vi "Vision Processing.vi"(4 "error in (no error)":errorcluster, 7 "Image Size":T9=enum."320x240") -> ()   [LabVIEW 2015]
doc: "This VI runs in parallel to other tasks. It gets images from the camera, processes them for color or shape and use that information to affect robot behavior."
uses:
  <vilib>/Rock Robotics/WPI/Camera/WPI_CameraImageSize.ctl
  <vilib>/vision/Measure.llb/Straight Edge Options.ctl
  <vilib>/vision/Measure.llb/Straight Edge Process.ctl
  <vilib>/vision/Measure.llb/Edge Options.ctl
  <vilib>/vision/Measure.llb/Edge Polarity.ctl
  <vilib>/Rock Robotics/WPI/Camera/WPI_CameraWhite Balance Values.ctl
  <vilib>/Rock Robotics/WPI/Camera/WPI_CameraExposure Values.ctl
  <vilib>/Rock Robotics/WPI/Camera/WPI_CameraFrameRate.ctl
  Robot Global Data.vi
  <vilib>/vision/NI_Vision_Development_Module.lvlib
panel:
  in  "Options":T3={"Search Direction"=0, "Edge Options"={"Edge Polarity"=0, "Kernel Size"=3, "Width"=3, "Minimum Edge Strength"=10.0, "Interpolation Type"=enum."Bilinear Fixed", "Data Processing Method"=enum."Average"}, "Show Search Area"=FALSE, "Show Search Lines"=FALSE, "Show Edges Found"=FALSE, "Show Result"=TRUE, "Search Area Color"=65280, "Search Lines Color"=255, "Edge Locations Color"=16776960, "Result Color"=16711680, "Overlay Group Name"=""} {"Edge Options"."Edge Polarity" items=["All Edges", "Rising Edges", "Falling Edges"]; "Edge Options"."Minimum Edge Strength" format="%.2f"; "Edge Options"."Width" step=2; "Edge Options"."Kernel Size" step=2; "Search Direction" items=["Left to Right", "Right to Left", "Top to Bottom", "Bottom to Top"]}
  out "Image Dst Out":T4(plugin-control)
  out "Corner Point Coordinates[0]":cluster{"X":sgl, "Y":sgl}
  out "Point2 (Pixels)":cluster{"X":sgl, "Y":sgl}
  out "Point1 (Pixels)":cluster{"X":sgl, "Y":sgl}
  in  "Line Fit Options":T5={"Number of Lines"=1, "Type"=enum."First Edge Rake", "Min. Score"=10.0, "Max. Score"=1000.0, "Orientation"=0.0, "Angle Range"=45.0, "Angle Tolerance"=1.0, "Step Size"=7, "Min. SNR (db)"=0.0, "Min. Points (%)"=25.0, "Hough Iterations"=5} {"Min. Points (%)" min=0.0 max=100.0; "Min. SNR (db)" min=0.0; "Max. Score" min=0.0 max=1024.0; "Min. Score" min=0.0 max=1024.0 step=1.0}
  in  "Coordinate System":T7 {"Measurement System"."Axis Reference" items=["Direct", "Indirect"]; "Measurement System"."Angle (deg)" format="%.2f"; "Measurement System"."Origin"."Y" format="%.2f"; "Measurement System"."Origin"."X" format="%.2f"; "Reference System"."Axis Reference" items=["Direct", "Indirect"]; "Reference System"."Angle (deg)" format="%.2f"; "Reference System"."Origin"."Y" format="%.2f"; "Reference System"."Origin"."X" format="%.2f"}
  in  "ROI Descriptor":T8 {"Contours"."Type" items=["No Selection", "Point", "Line", "Rectangle", "Oval", "Polygon", "Free", "Annulus", "Unused2", "Unused3", "Broken Line", "Free Hand Line", "Rotated Rectangle"]}
  out "Center of Mass":cluster{"X":dbl, "Y":dbl}
  out "Calibration Valid":bool[](array[boolean])
  out "max index(es)":i32[](array[numeric])
  out "max value":u8
  in  "Range":cluster{"Lower value":i32, "Upper value":i32}={"Lower value"=240, "Upper value"=255}
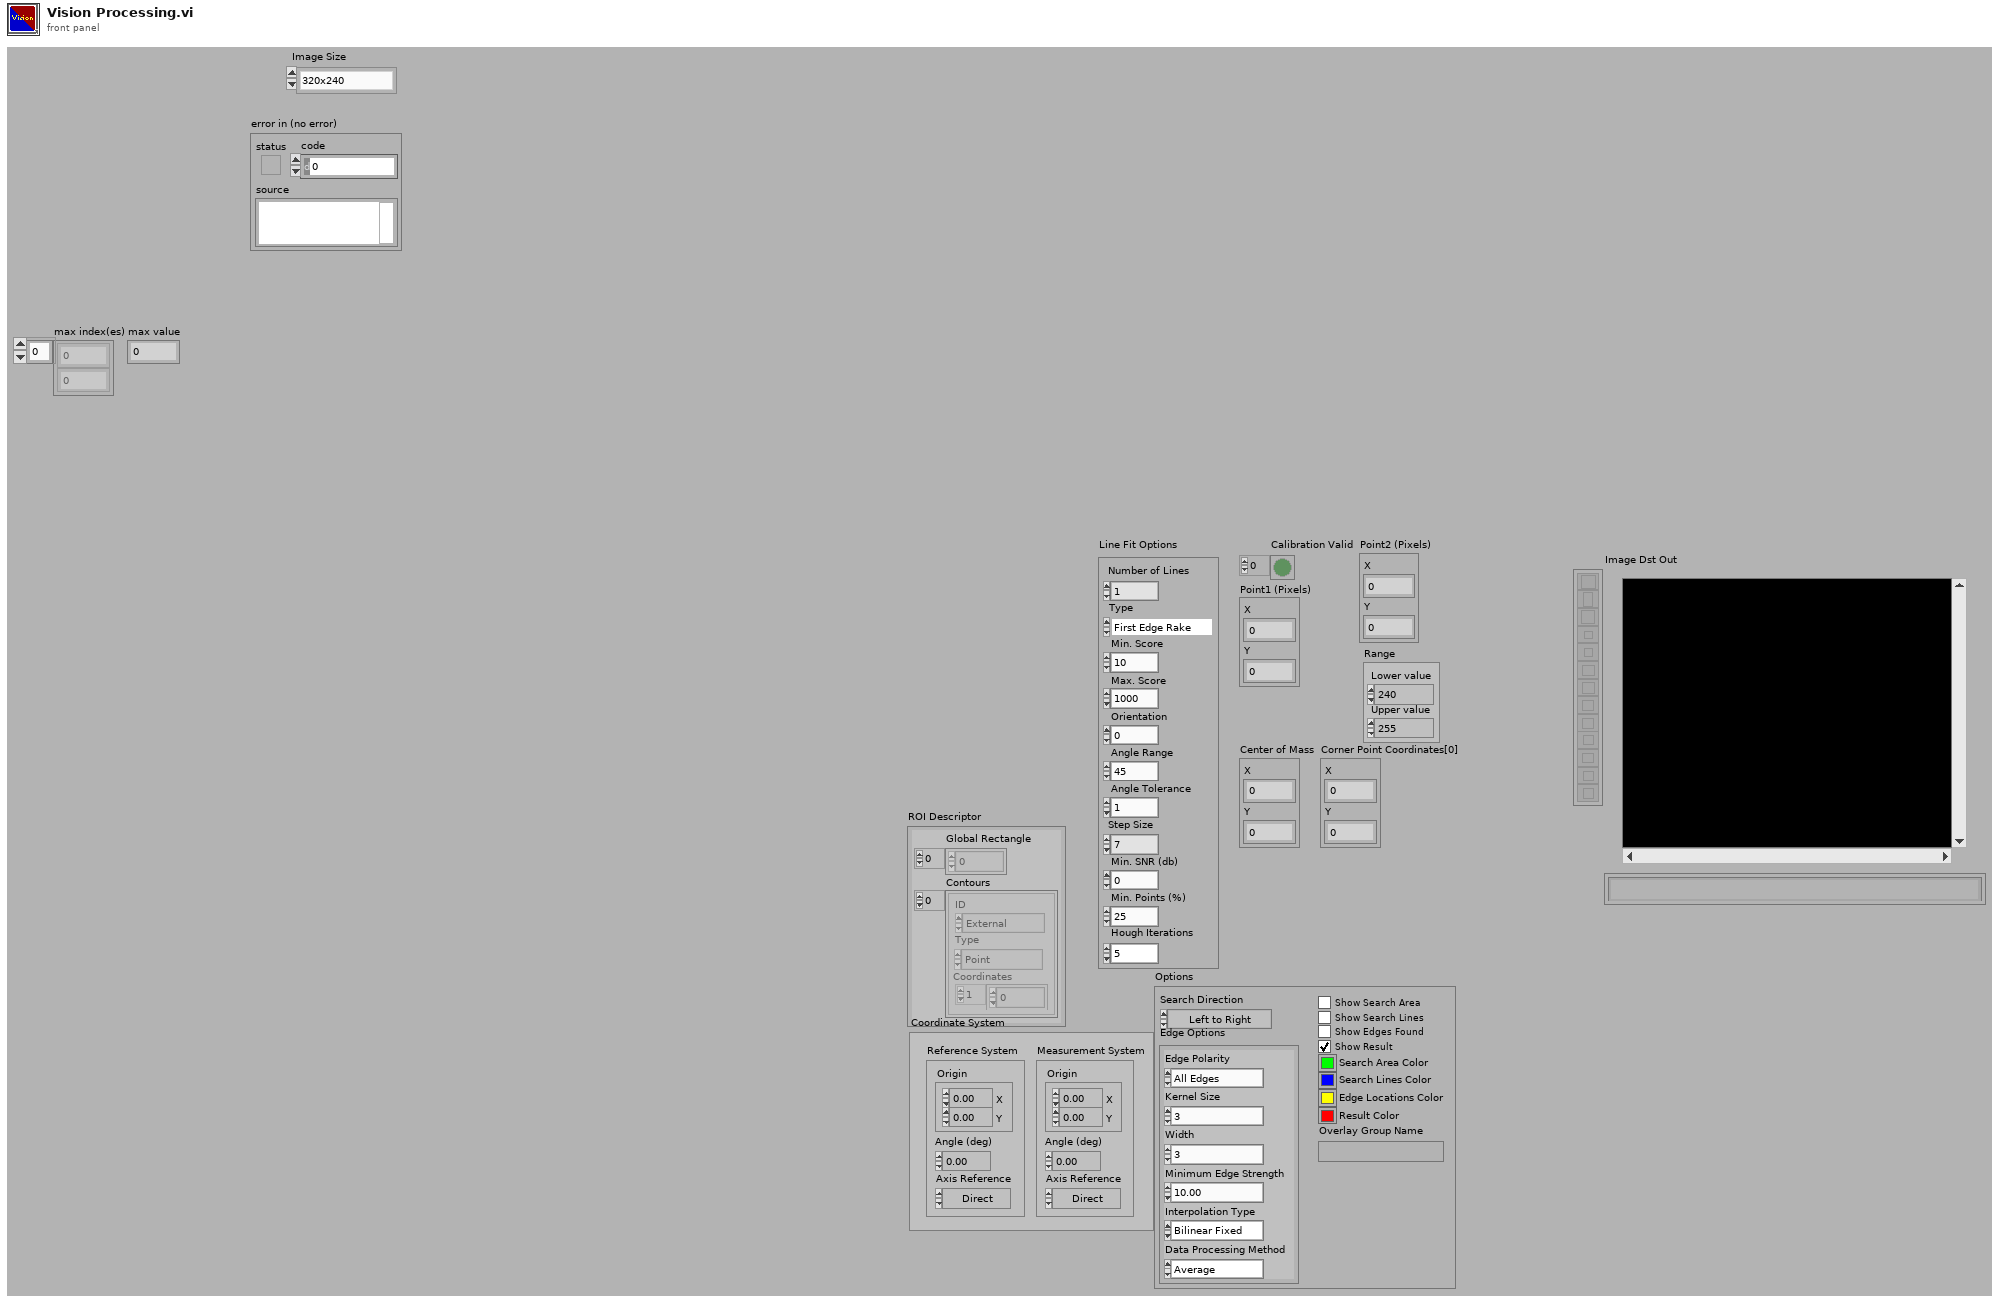
[diagram p1: front panel]
types:
  T1 = typedef "Edge Options.ctl" = cluster{"Edge Polarity":T2, "Kernel Size":u32, "Width":u32, "Minimum Edge Strength":sgl, "Interpolation Type":enum32{"Zero Order", "Bilinear", "Quadratic", "Cubic", "Bilinear Fixed"}, "Data Processing Method":enum32{"Average", "Median"}}
  T2 = typedef "Edge Polarity.ctl" = u32
  T3 = cluster{"Search Direction":u32, "Edge Options":T1, "Show Search Area":bool, "Show Search Lines":bool, "Show Edges Found":bool, "Show Result":bool, "Search Area Color":u32, "Search Lines Color":u32, "Edge Locations Color":u32, "Result Color":u32, "Overlay Group Name":string}
  T4 = typedef "IMAQ Image.ctl" = refnum<image>
  T5 = typedef "Straight Edge Options.ctl" = cluster{"Number of Lines":i32, "Type":T6, "Min. Score":dbl, "Max. Score":dbl, "Orientation":dbl, "Angle Range":dbl, "Angle Tolerance":dbl, "Step Size":u32, "Min. SNR (db)":dbl, "Min. Points (%)":dbl, "Hough Iterations":i32}
  T6 = typedef "Straight Edge Process.ctl" = enum32{"First Edge Rake", "Best Edge Rake", "Hough Edge Rake", "First Edge Projection", "Best Edge Projection"}
  T7 = typedef "IMAQ Coordinate System" = cluster{"Reference System":cluster{"Origin":cluster{"X":sgl, "Y":sgl}, "Angle (deg)":sgl, "Axis Reference":u32}, "Measurement System":cluster{"Origin":cluster{"X":sgl, "Y":sgl}, "Angle (deg)":sgl, "Axis Reference":u32}}
  T8 = cluster{"Global Rectangle":i32[], "Contours":cluster{"ID":enum32{"External", "Internal"}, "Type":u32, "Coordinates":i32[]}[]}
  T9 = typedef "WPI_CameraImageSize.ctl" = enum16{"640x480", "320x240", "160x120", "Custom"}
  T10 = typedef "Image Type" = u32
  T11 = typedef "WPI_CameraFrameRate.ctl" = u32
  T12 = typedef "WPI_CameraExposure Values.ctl" = enum16{"Auto", "Flicker-free 50 Hz", "Flicker-free 60 Hz", "Hold current", "Custom"}
  T13 = typedef "WPI_CameraWhite Balance Values.ctl" = enum16{"Auto", "Fixed indoor", "Fixed outdoor 1", "Fixed outdoor 2", "Fixed fluorescent 1", "Fixed fluorescent 2", "Hold current", "Custom"}
  T14 = typedef "WPI_CameraDevRef.ctl" = cluster{"Camera Address":string, "CameraStatus":errorcluster}
  T15 = enum32{"AutoM", "Close", "Dilate", "Erode", "Gradient", "Gradient out", "Gradient in", "Hit miss", "Open", "PClose", "POpen", "Thick", "Thin"}
  T16 = cluster{"Area":dbl, "Number of Holes":dbl, "Bounding Rect":cluster{"Left":dbl, "Top":dbl, "Right":dbl, "Bottom":dbl}, "Center of Mass":cluster{"X":dbl, "Y":dbl}, "Orientation":dbl, "Dimensions":cluster{"Width":dbl, "Height":dbl}}[]
  T17 = cluster{"Point1 (Pixels)":cluster{"X":sgl, "Y":sgl}, "Point2 (Pixels)":cluster{"X":sgl, "Y":sgl}, "Point1 (Real-World)":cluster{"X":sgl, "Y":sgl}, "Point2 (Real-World)":cluster{"X":sgl, "Y":sgl}, "Angle (Pixel)":dbl, "Angle (Real-World)":dbl, "Score":dbl, "Straightness":dbl, "Average SNR (db)":dbl, "Calibration Valid":bool}[]
  T18 = cluster{"Particle Reports (Pixels)[0]":cluster{"Area":dbl, "Number of Holes":dbl, "Bounding Rect":cluster{"Left":dbl, "Top":dbl, "Right":dbl, "Bottom":dbl}, "Center of Mass":cluster{"X":dbl, "Y":dbl}, "Orientation":dbl, "Dimensions":cluster{"Width":dbl, "Height":dbl}}, "Particle Reports (Pixels)[1]":cluster{"Area":dbl, "Number of Holes":dbl, "Bounding Rect":cluster{"Left":dbl, "Top":dbl, "Right":dbl, "Bottom":dbl}, "Center of Mass":cluster{"X":dbl, "Y":dbl}, "Orientation":dbl, "Dimensions":cluster{"Width":dbl, "Height":dbl}}, "Particle Reports (Pixels)[2]":cluster{"Area":dbl, "Number of Holes":dbl, "Bounding Rect":cluster{"Left":dbl, "Top":dbl, "Right":dbl, "Bottom":dbl}, "Center of Mass":cluster{"X":dbl, "Y":dbl}, "Orientation":dbl, "Dimensions":cluster{"Width":dbl, "Height":dbl}}, "Particle Reports (Pixels)[3]":cluster{"Area":dbl, "Number of Holes":dbl, "Bounding Rect":cluster{"Left":dbl, "Top":dbl, "Right":dbl, "Bottom":dbl}, "Center of Mass":cluster{"X":dbl, "Y":dbl}, "Orientation":dbl, "Dimensions":cluster{"Width":dbl, "Height":dbl}}, "Particle Reports (Pixels)[4]":cluster{"Area":dbl, "Number of Holes":dbl, "Bounding Rect":cluster{"Left":dbl, "Top":dbl, "Right":dbl, "Bottom":dbl}, "Center of Mass":cluster{"X":dbl, "Y":dbl}, "Orientation":dbl, "Dimensions":cluster{"Width":dbl, "Height":dbl}}, "Particle Reports (Pixels)[5]":cluster{"Area":dbl, "Number of Holes":dbl, "Bounding Rect":cluster{"Left":dbl, "Top":dbl, "Right":dbl, "Bottom":dbl}, "Center of Mass":cluster{"X":dbl, "Y":dbl}, "Orientation":dbl, "Dimensions":cluster{"Width":dbl, "Height":dbl}}, "Particle Reports (Pixels)[6]":cluster{"Area":dbl, "Number of Holes":dbl, "Bounding Rect":cluster{"Left":dbl, "Top":dbl, "Right":dbl, "Bottom":dbl}, "Center of Mass":cluster{"X":dbl, "Y":dbl}, "Orientation":dbl, "Dimensions":cluster{"Width":dbl, "Height":dbl}}, "Particle Reports (Pixels)[7]":cluster{"Area":dbl, "Number of Holes":dbl, "Bounding Rect":cluster{"Left":dbl, "Top":dbl, "Right":dbl, "Bottom":dbl}, "Center of Mass":cluster{"X":dbl, "Y":dbl}, "Orientation":dbl, "Dimensions":cluster{"Width":dbl, "Height":dbl}}, "Particle Reports (Pixels)[8]":cluster{"Area":dbl, "Number of Holes":dbl, "Bounding Rect":cluster{"Left":dbl, "Top":dbl, "Right":dbl, "Bottom":dbl}, "Center of Mass":cluster{"X":dbl, "Y":dbl}, "Orientation":dbl, "Dimensions":cluster{"Width":dbl, "Height":dbl}}}
  T19 = cluster{"Corner Point Coordinates[0]":cluster{"X":sgl, "Y":sgl}, "Corner Point Coordinates[1]":cluster{"X":sgl, "Y":sgl}, "Corner Point Coordinates[2]":cluster{"X":sgl, "Y":sgl}, "Corner Point Coordinates[3]":cluster{"X":sgl, "Y":sgl}, "Corner Point Coordinates[4]":cluster{"X":sgl, "Y":sgl}, "Corner Point Coordinates[5]":cluster{"X":sgl, "Y":sgl}, "Corner Point Coordinates[6]":cluster{"X":sgl, "Y":sgl}, "Corner Point Coordinates[7]":cluster{"X":sgl, "Y":sgl}, "Corner Point Coordinates[8]":cluster{"X":sgl, "Y":sgl}}
  T20 = cluster{"Point1 (Pixels)":cluster{"X":sgl, "Y":sgl}, "Point2 (Pixels)":cluster{"X":sgl, "Y":sgl}, "Point1 (Real-World)":cluster{"X":sgl, "Y":sgl}, "Point2 (Real-World)":cluster{"X":sgl, "Y":sgl}, "Angle (Pixel)":dbl, "Angle (Real-World)":dbl, "Score":dbl, "Straightness":dbl, "Average SNR (db)":dbl, "Calibration Valid":bool}
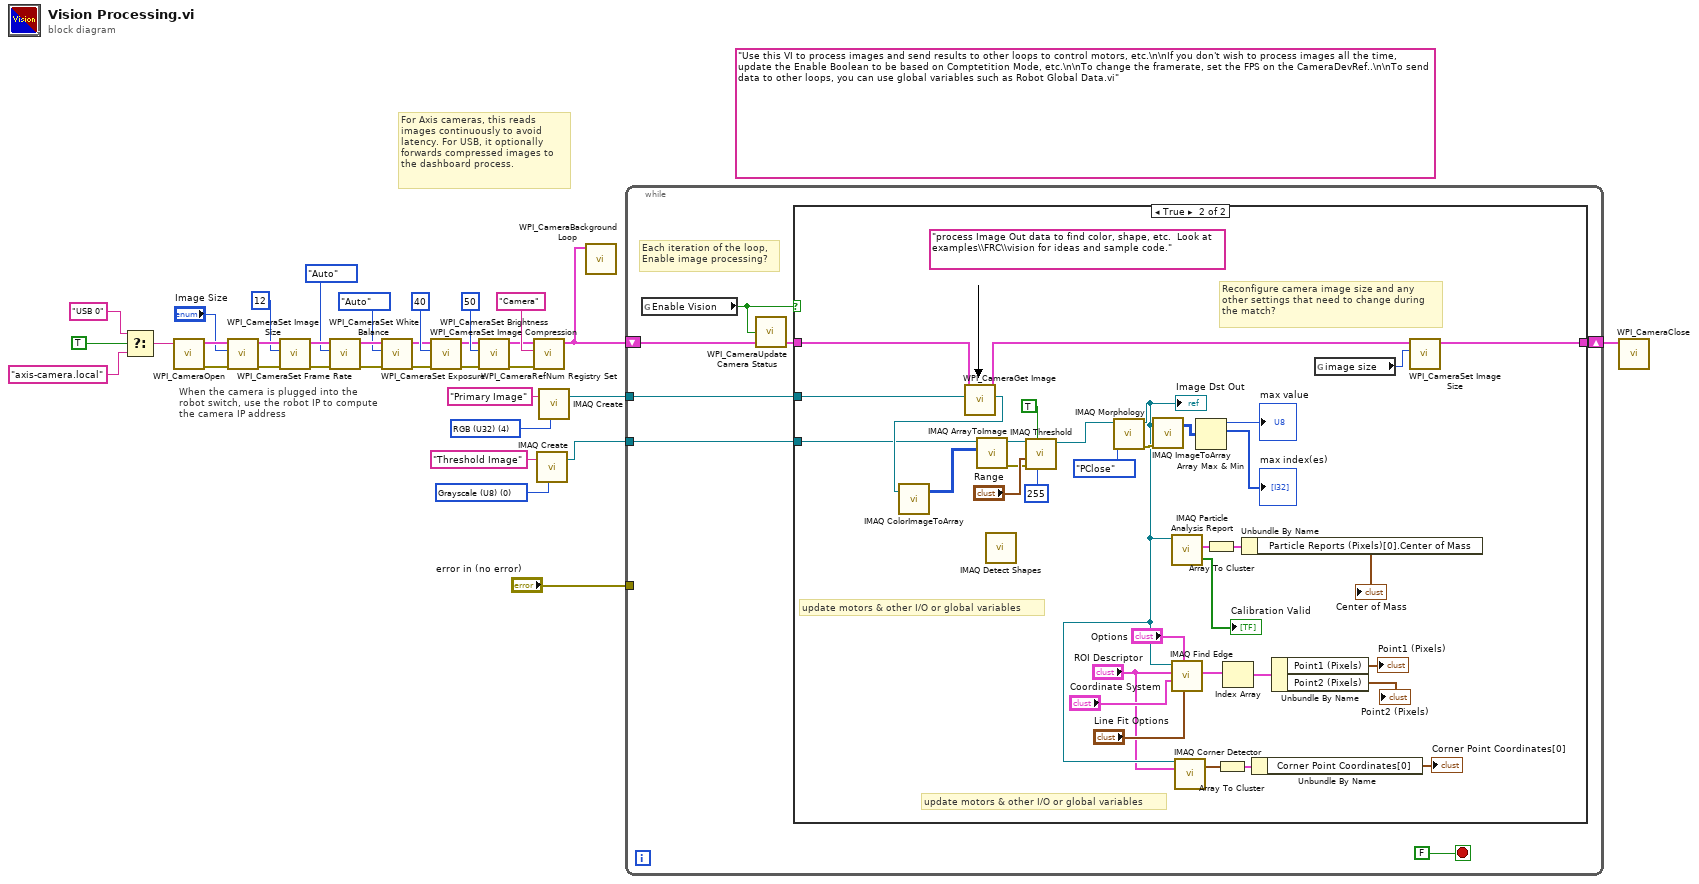
[diagram p0: block diagram]
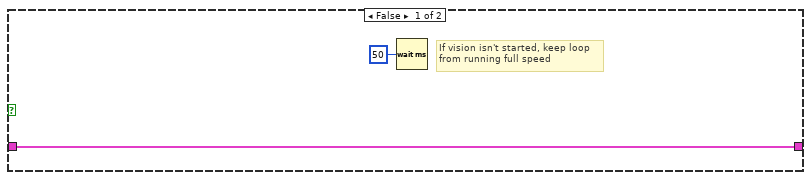
[diagram p2: hidden frame]
diagram:
  w3 = T10 0 items=["Grayscale (U8)", "Grayscale (I16)", "Grayscale (SGL)", "Complex (CSG)", "RGB (U32)", "HSL (U32)", "RGB (U64)", "Grayscale (U16)"] ("Image Type")
  (unwired) "Use this VI to process images and send results to other loops to control motors, etc.\n\nIf you don't wish to process images all the time, update the Enable Boolean to be based on Comptetition Mode, etc.\n\nTo change the framerate, set the FPS on the CameraDevRef..\n\nTo send data to other loops, you can use global variables such as Robot Global Data.vi"
  w34 = T10 4 items=["Grayscale (U8)", "Grayscale (I16)", "Grayscale (SGL)", "Complex (CSG)", "RGB (U32)", "HSL (U32)", "RGB (U64)"] ("Image Type")
  # "When the camera is plugged into the\nrobot switch, use the robot IP to compute\nthe camera IP address"
  # "For Axis cameras, this reads\nimages continuously to avoid\nlatency. For USB, it optionally\nforwards compressed images to\nthe dashboard process."
  n1 = Select(t="USB 0" ("format string"), s=TRUE ("dot notation? (F)"), f="axis-camera.local" ("format string")) -> (s? t:f=w5:string)
  n2 = call <vilib>:"WPI_CameraOpen.vi"("Camera Address"=w5) -> ("error out"=w22:errorcluster, "CameraDevRef"=w23:T14)  [unwired: 1 in, 8 out]
  n3 = call <vilib>:"WPI_CameraSet Image Size.vi"("error in (no error)"=w22, "Image Size"="Image Size", "CameraDevRef"=w23) -> ("error out"=w21:errorcluster, "CameraDevRef Out"=w24:T14)  [unwired: 1 in, 6 out]
  n4 = call <vilib>:"WPI_CameraSet Frame Rate.vi"("error in (no error)"=w21, "Frame Rate (fps)"=T11 12, "CameraDevRef"=w24) -> ("error out"=w20:errorcluster, "CameraDevRef Out"=w26:T14)  [unwired: 7 out]
  n5 = call <vilib>:"WPI_CameraSet White Balance.vi"("error in (no error)"=w20, "White Balance"=WPI_CameraWhite_Balance_Values."Auto", "CameraDevRef"=w26) -> ("error out"=w19:errorcluster, "CameraDevRef Out"=w25:T14)  [unwired: 1 in, 6 out]
  n6 = call <vilib>:"WPI_CameraSet Exposure.vi"("error in (no error)"=w19, "Exposure"=WPI_CameraExposure_Values."Auto", "CameraDevRef"=w25) -> ("error out"=w18:errorcluster, "CameraDevRef Out"=w28:T14)  [unwired: 1 in, 6 out]
  n7 = call <vilib>:"WPI_CameraSet Image Compression.vi"("error in (no error)"=w18, "Compression"=40, "CameraDevRef"=w28) -> ("error out"=w17:errorcluster, "CameraDevRef Out"=w27:T14)  [unwired: 7 out]
  n8 = call <vilib>:"WPI_CameraSet Brightness.vi"("error in (no error)"=w17, "Brightness"=50, "CameraDevRef"=w27) -> ("error out"=w15:errorcluster, "CameraDevRef Out"=w16:T14)  [unwired: 7 out]
  n9 = call <vilib>:"WPI_CameraRefNum Registry Set.vi"("error in (no error)"=w15, "refnum name"="Camera", "CameraDevRef"=w16) -> ("CameraDevRef"=w11:T14)  [unwired: 1 in, 7 out]
  n10 = call "IMAQ Create"("Image Name"="Threshold Image", "Image Type"=w3) -> ("New Image"=w1:T4)  [unwired: 3 in, 1 out]
  n11 = call "IMAQ Create"("Image Name"="Primary Image", "Image Type"=w34) -> ("New Image"=w32:T4)  [unwired: 2 in, 2 out]
  n12 = call <vilib>:"WPI_CameraBackground Loop.vi"("CameraDevRef"=w11) -> ()  [unwired: 11 in]
  n13 = while {
    shift-right: [w40] -> w9
    shift-left: w11 -> [w38]
    tunnel: w32 -> [w39]
    tunnel: "error in (no error)" -> [_]
    tunnel: w1 -> [w35]
    stop <- FALSE stop-if-true
    # "Each iteration of the loop,\nEnable image processing?"
    n14 = global read "Robot Global Data.vi" "Enable Vision"() -> (w36:bool)
    n15 = call <vilib>:"WPI_CameraUpdate Camera Status.vi"("CameraDevRef In"=w38, "Enable Vision"=w36) -> ("CameraDevRef Out"=w37:T14)  [unwired: 3 in]
    n16 = case shown="True" w36 {
      tunnel: w39 -> [_ w77]
      tunnel: [w43 w78] -> w40
      tunnel: w37 -> [w43 w75]
      tunnel: w35 -> [_ w44]
      frame False {
        # "If vision isn't started, keep loop\nfrom running full speed"
        n17 = Wait (ms)(milliseconds to wait=u32 50) -> ()  [unwired: 1 out]
      }
      frame True {
        (unwired) "process Image Out data to find color, shape, etc.  Look at examples\\FRC\\vision for ideas and sample code."
        # "update motors & other I/O or global variables"
        # "update motors & other I/O or global variables"
        # "Reconfigure camera image size and any\nother settings that need to change during\nthe match?"
        n18 = call <vilib>:"WPI_CameraGet Image.vi"("Image"=w77, "CameraDevRef"=w75) -> ("Image Out"=w45:T4, "CameraDevRef Out"=w74:T14)  [unwired: 1 in, 7 out]
        n19 = call "IMAQ ColorImageToArray"("Image"=w45) -> ("Image Pixels (U32)"=w73:u32[][])  [unwired: 3 in, 2 out]
        n20 = call "IMAQ ArrayToImage"("Image Pixels (U8)"=w73, "Image"=w44) -> ("error out"=w67:errorcluster, "Image Out"=w68:T4)  [unwired: 8 in]
        n21 = call-poly "IMAQ Detect Shapes"() -> ()  [unwired: 9 in, 3 out]
        n22 = call "IMAQ Threshold"("Replace Value"=255, "Keep/Replace Value (Replace)"=TRUE, "error in (no error)"=w67, "Range"="Range", "Image Src"=w68) -> ("Image Dst Out"=w62:T4)  [unwired: 5 in, 1 out]
        n23 = call "IMAQ Morphology"("Operation"=T15."PClose", "Image Src"=w62) -> ("error out"=w64:errorcluster, "Image Dst Out"=w48:T4)  [unwired: 8 in]
        "Image Dst Out" <- w48
        n24 = call "IMAQ ImageToArray"("error in (no error)"=w64, "Image"=w48) -> ("Image Pixels (I16)"=w63:i16[][])  [unwired: 2 in, 4 out]
        n25 = call "IMAQ Particle Analysis Report"("Image"=w48) -> ("Particle Reports (Pixels)"=w61:T16, "Calibration Valid"=→"Calibration Valid":bool[])  [unwired: 5 in, 4 out]
        n26 = call "IMAQ Find Edge"("Line Fit Options"="Line Fit Options", "Options"="Options", "Coordinate System"="Coordinate System", "ROI Descriptor"="ROI Descriptor", "Image"=w48) -> ("Straight Edges"=w55:T17)  [unwired: 3 in, 3 out]
        n27 = call "IMAQ Corner Detector"("Image"=w48, "ROI Descriptor"="ROI Descriptor") -> ("Corner Point Coordinates"=w51:cluster{"X":sgl, "Y":sgl}[])  [unwired: 8 in, 5 out]
        n28 = Array Max & Min(array=w63) -> (max value=→"max value":i16, max index (indices)=→"max index(es)":i32[])  [unwired: 2 out]
        n29 = Array To Cluster(array=w61) -> (cluster=w60:T18)
        n30 = Array To Cluster(array=w51) -> (cluster=w50:T19)
        n31 = Index Array(array=w55) -> (element=w54:T20)  [unwired: 1 in]
        n32 = Unbundle By Name(w60) -> ("Particle Reports (Pixels)[0].Center of Mass"=→"Center of Mass":cluster{"X":dbl, "Y":dbl})
        n33 = Unbundle By Name(w50) -> ("Corner Point Coordinates[0]"=→"Corner Point Coordinates[0]":cluster{"X":sgl, "Y":sgl})
        n34 = Unbundle By Name(w54) -> ("Point1 (Pixels)"=→"Point1 (Pixels)":cluster{"X":sgl, "Y":sgl}, "Point2 (Pixels)"=→"Point2 (Pixels)":cluster{"X":sgl, "Y":sgl})
        n35 = global read "Robot Global Data.vi" "image size"() -> (w76:T9)
        n36 = call <vilib>:"WPI_CameraSet Image Size.vi"("Image Size"=w76, "CameraDevRef"=w74) -> ("CameraDevRef Out"=w78:T14)  [unwired: 2 in, 7 out]
      }
    }
  }
  n37 = call <vilib>:"WPI_CameraClose.vi"("CameraDevRef"=w9) -> ()  [unwired: 1 in, 10 out]
